vi "Agilent 34970 Array to Scan List.vi"(11 "Agilent Channels (Temperature TC)":string[](array[string])) -> (3 "Agilent Scan List":string)   [LabVIEW 2018]
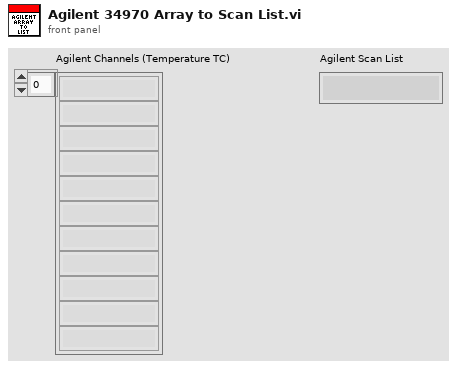
[diagram p1: front panel]
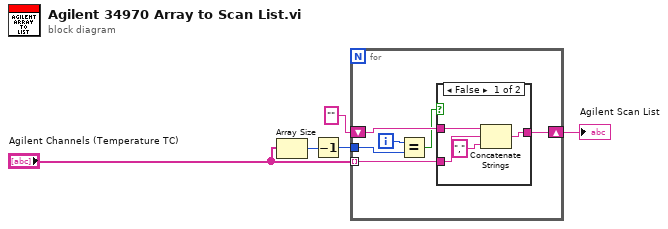
[diagram p0: block diagram]
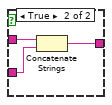
[diagram p2: hidden frame]
diagram:
  n1 = Array Size(array="Agilent Channels (Temperature TC)") -> (size(s)=w2:i32)
  n2 = Decrement(x=w2) -> (x-1=w1:i32)
  n3 = for {
    shift-right: [w9] -> w5
    shift-left: "" -> [w11]
    tunnel: "Agilent Channels (Temperature TC)" -> [w10] mode=indexing
    tunnel: w1 -> [w7]
    i -> [w8]
    n4 = Equal?(x=w8, y=w7) -> (x = y?=w6:bool)
    n5 = case shown="False" w6 {
      tunnel: w11 -> [w15 w18]
      tunnel: w10 -> [w14 w16]
      tunnel: [w12 w17] -> w9
      frame False {
        n6 = Concatenate Strings(w15, w14, ",") -> (w12:string)
      }
      frame True {
        n7 = Concatenate Strings(w18, w16) -> (w17:string)
      }
    }
  }
  "Agilent Scan List" <- w5
